vi "flushQueue.vi"(8 "error in (no error)":errorcluster, 11 "MissionQueue in":refnum<class "MissionQueue.lvclass">) -> (0 "error out":errorcluster, 2 "remaining elements":refnum<class "GenericMission.lvclass">[](array[class]), 3 "MissionQueue out":refnum<class "MissionQueue.lvclass">)   [LabVIEW 2011, in "MissionQueue.lvclass"]
uses:
  MissionQueue.lvclass
  Missions/GenericMission/GenericMission.lvclass
  MissionQueue.lvclass/MissionQueue.ctl
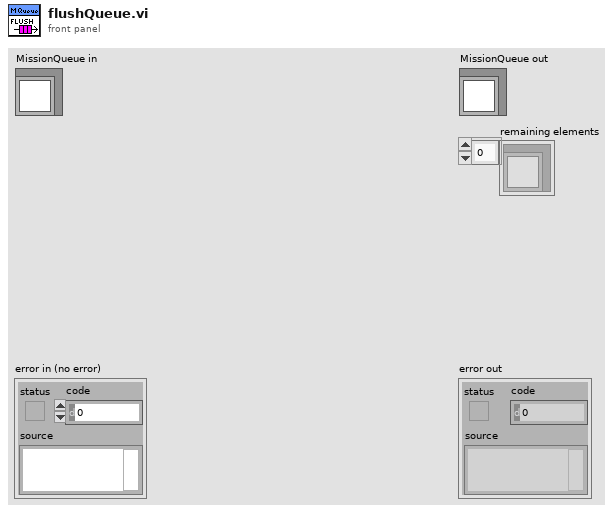
[diagram p1: front panel]
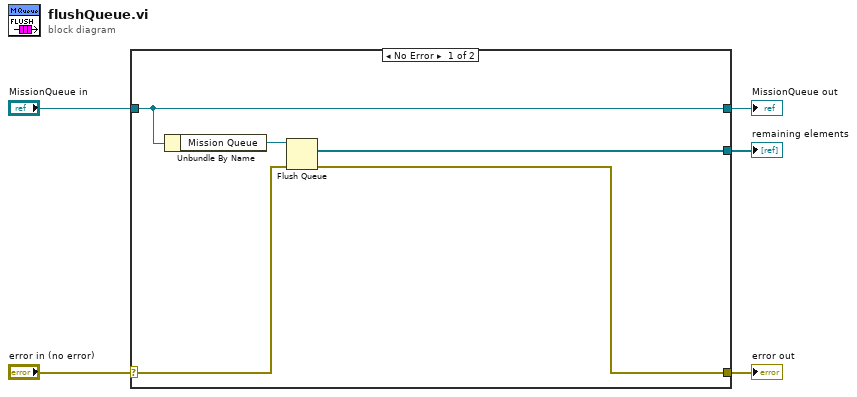
[diagram p0: block diagram]
diagram:
  n1 = case shown="No Error" "error in (no error)" {
    selector: "error in (no error)" -> [w9 w12]
    tunnel: [w8 w12] -> w4
    tunnel: [w7 w11] -> w2
    tunnel: "MissionQueue in" -> [w7 w11]
    tunnel: [w6 _] -> w1
    frame No Error {
      n2 = Unbundle By Name(w7) -> ("Mission Queue"=w10:refnum<queue>)
      n3 = Flush Queue(queue=w10, error in (no error)=w9) -> (remaining elements=w6:refnum<class "GenericMission.lvclass">[], error out=w8:errorcluster)  [unwired: 1 out]
    }
    frame Error {
    }
  }
  "error out" <- w4
  "MissionQueue out" <- w2
  "remaining elements" <- w1
